vi "SetAxisParameter.vi"(8 "error in (no error)":errorcluster, 11 "ZanClass in":refnum<class "ZanClass.lvclass">) -> (0 "error out":errorcluster, 3 "ZanClass out":refnum<class "ZanClass.lvclass">)   [LabVIEW 2019, in "ZanClass.lvclass"]
uses:
  ZanClass.lvclass
  LLB/zmotion/zaux/zauxdll.lvlib
  Ctrl/CardTypr.ctl
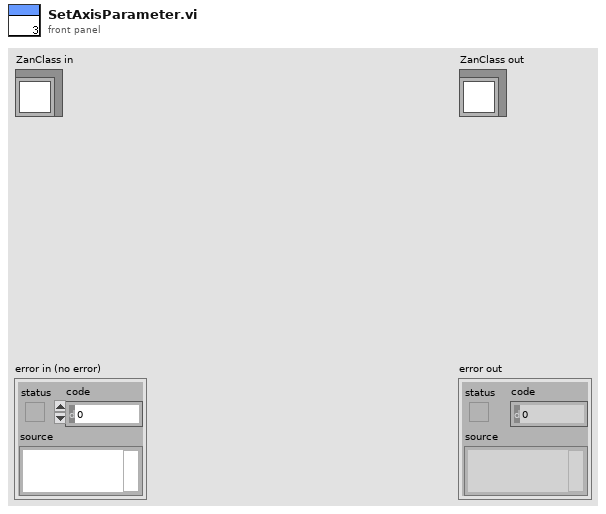
[diagram p1: front panel]
types:
  T1 = typedef "IO Card_Type.ctl" = enum16{"None", "Unidaq32", "6480", "2410C-64", "Zan", "DMC1000B", "16InOut", "Robot", "DMC3600"}
  T2 = cluster{"SetAType":i32, "SetUnit":sgl, "SetInvertStep":i32, "SetFwdIn":i32, "SetDatumIn":i32, "SetRevIn":i32, "SetAlmIn":i32}[]
  T3 = typedef "CardTypr.ctl" = enum16{"DMC2410", "DMC6480", "ZMotion", "KingServo RSCmd", "Zmotion2"}
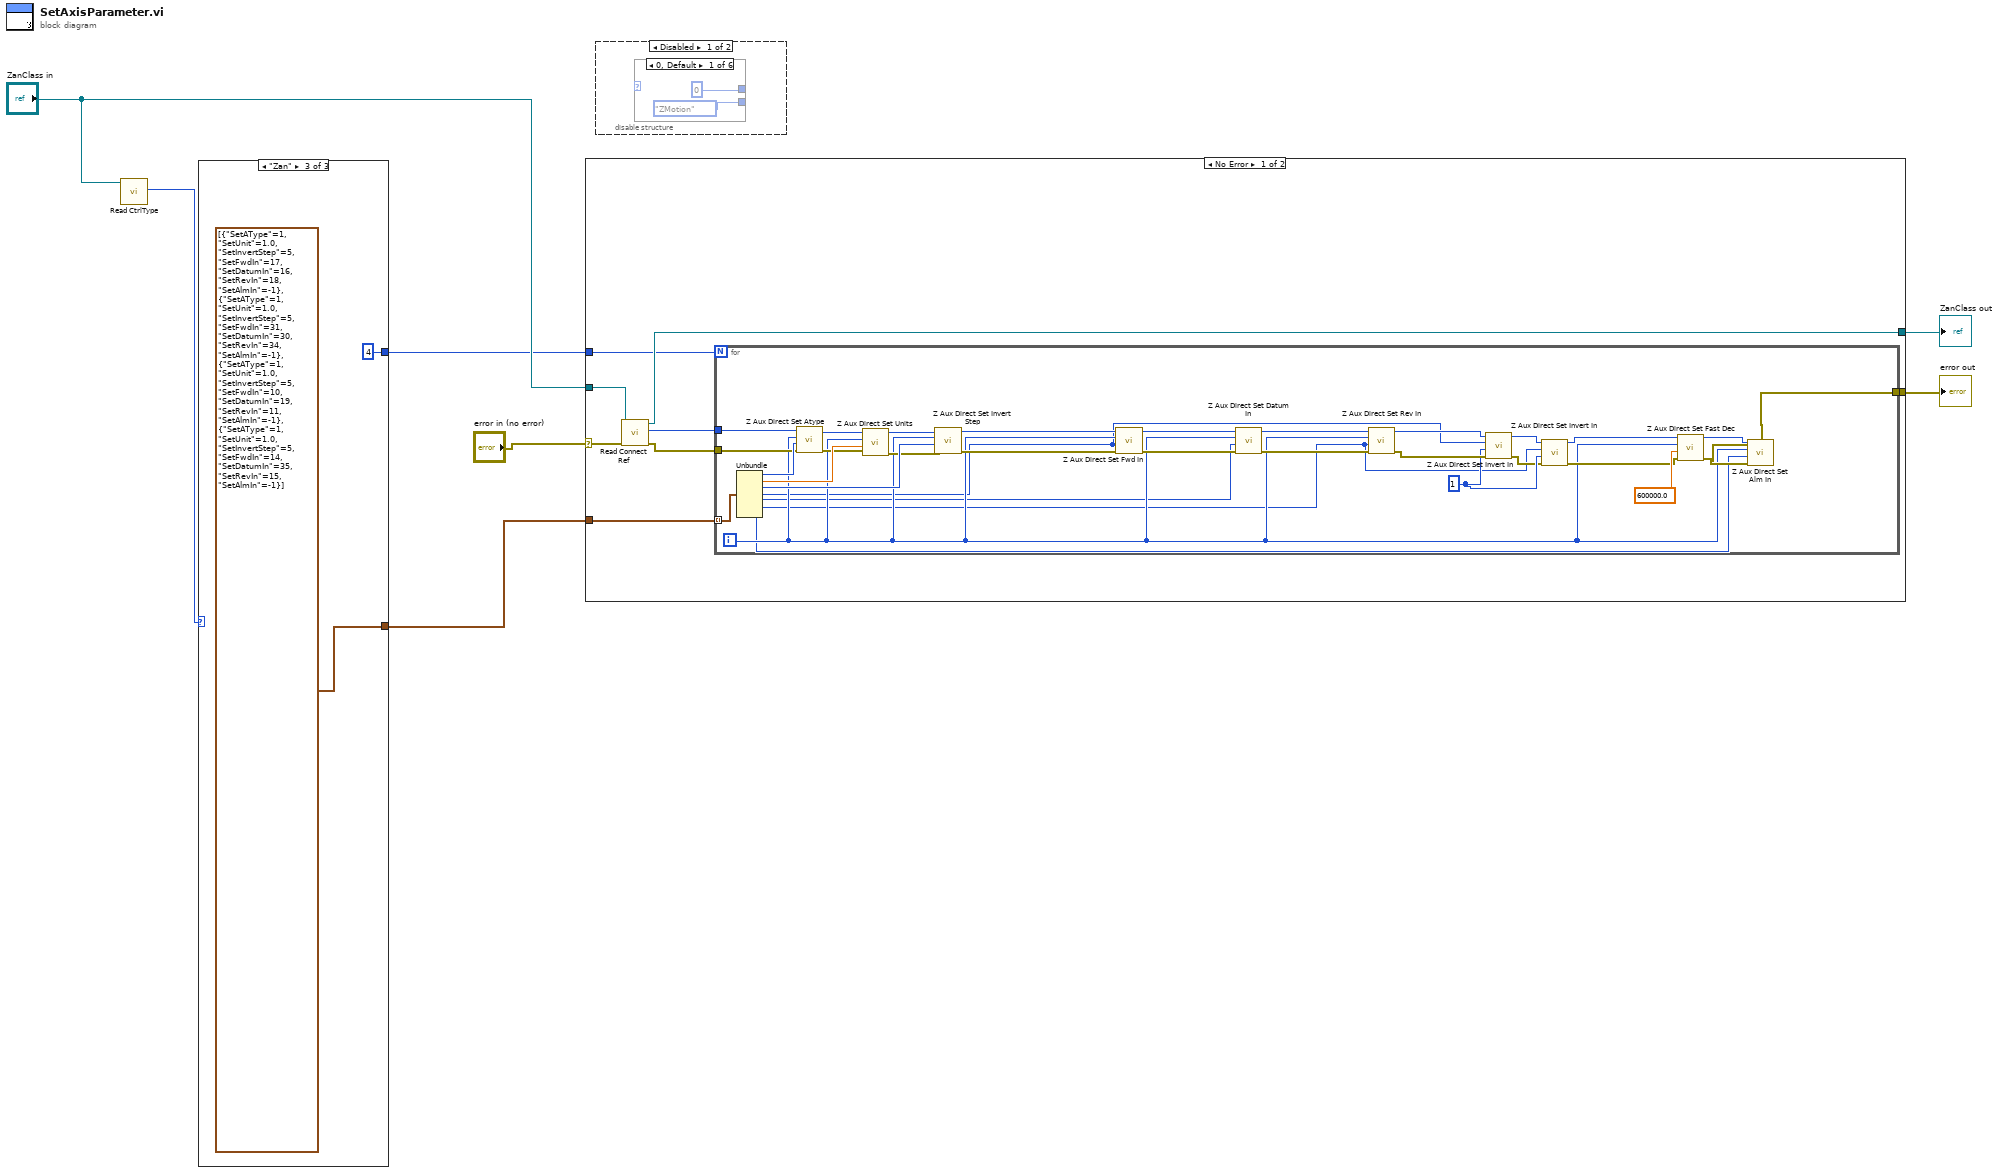
[diagram p0: block diagram]
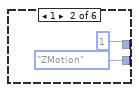
[diagram p2: hidden frame]
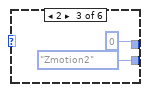
[diagram p3: hidden frame]
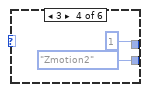
[diagram p4: hidden frame]
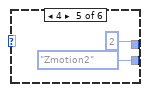
[diagram p5: hidden frame]
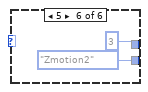
[diagram p6: hidden frame]
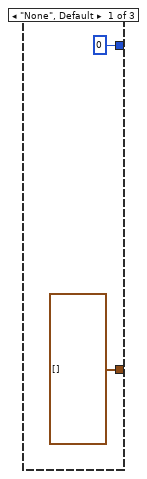
[diagram p8: hidden frame]
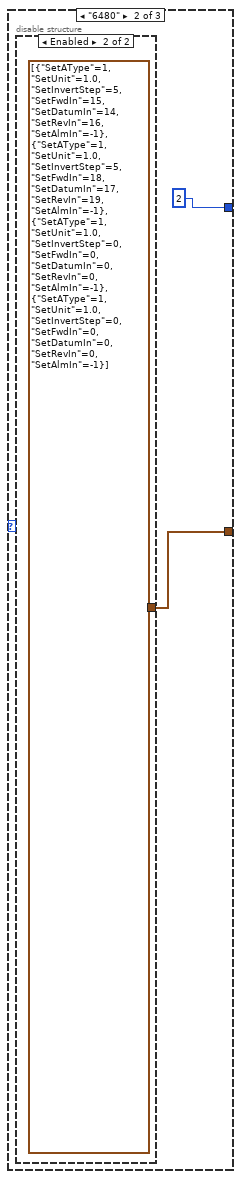
[diagram p9: hidden frame]
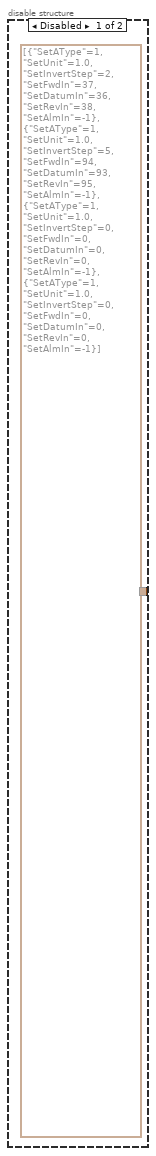
[diagram p10: hidden frame]
diagram:
  n1 = call-dynamic "Read CtrlType.vi"("AxisCard in"="ZanClass in") -> ("IO Card Type"=w2:T1)  [unwired: 8 in, 2 out]
  n2 = case shown="\"Zan\"" w2 {
    tunnel: [T2 [] w11 T2 [{"SetAType"=1, "SetUnit"=1.0, "SetInvertStep"=5, "SetFwdIn"=17, "SetDatumIn"=16, "SetRevIn"=18, "SetAlmIn"=-1}, {"SetAType"=1, "SetUnit"=1.0, "SetInvertStep"=5, "SetFwdIn"=31, "SetDatumIn"=30, "SetRevIn"=34, "SetAlmIn"=-1}, {"SetAType"=1, "SetUnit"=1.0, "SetInvertStep"=5, "SetFwdIn"=10, "SetDatumIn"=19, "SetRevIn"=11, "SetAlmIn"=-1}, {"SetAType"=1, "SetUnit"=1.0, "SetInvertStep"=5, "SetFwdIn"=14, "SetDatumIn"=35, "SetRevIn"=15, "SetAlmIn"=-1}]] -> w6
    tunnel: [0 2 4] -> w1
    frame "None", Default {
    }
    frame "6480" {
      n3 = disable-structure shown="Enabled" {
        disable-tunnel: [T2 [{"SetAType"=1, "SetUnit"=1.0, "SetInvertStep"=2, "SetFwdIn"=37, "SetDatumIn"=36, "SetRevIn"=38, "SetAlmIn"=-1}, {"SetAType"=1, "SetUnit"=1.0, "SetInvertStep"=5, "SetFwdIn"=94, "SetDatumIn"=93, "SetRevIn"=95, "SetAlmIn"=-1}, {"SetAType"=1, "SetUnit"=1.0, "SetInvertStep"=0, "SetFwdIn"=0, "SetDatumIn"=0, "SetRevIn"=0, "SetAlmIn"=-1}, {"SetAType"=1, "SetUnit"=1.0, "SetInvertStep"=0, "SetFwdIn"=0, "SetDatumIn"=0, "SetRevIn"=0, "SetAlmIn"=-1}] T2 [{"SetAType"=1, "SetUnit"=1.0, "SetInvertStep"=5, "SetFwdIn"=15, "SetDatumIn"=14, "SetRevIn"=16, "SetAlmIn"=-1}, {"SetAType"=1, "SetUnit"=1.0, "SetInvertStep"=5, "SetFwdIn"=18, "SetDatumIn"=17, "SetRevIn"=19, "SetAlmIn"=-1}, {"SetAType"=1, "SetUnit"=1.0, "SetInvertStep"=0, "SetFwdIn"=0, "SetDatumIn"=0, "SetRevIn"=0, "SetAlmIn"=-1}, {"SetAType"=1, "SetUnit"=1.0, "SetInvertStep"=0, "SetFwdIn"=0, "SetDatumIn"=0, "SetRevIn"=0, "SetAlmIn"=-1}]] -> w11
        frame Disabled {
        }
        frame Enabled {
        }
      }
    }
    frame "Zan" {
    }
  }
  n4 = case shown="No Error" "error in (no error)" {
    selector: "error in (no error)" -> [w19 w56]
    tunnel: "ZanClass in" -> [w23 w57]
    tunnel: w6 -> [w21 _]
    tunnel: [w20 w57] -> w5
    tunnel: [w17 w56] -> w4
    tunnel: w1 -> [w16 _]
    frame No Error {
      n5 = call-dynamic "Read Connect Ref.vi"("error in (no error)"=w19, "ZanClass in"=w23) -> ("error out"=w18:errorcluster, "CardHandle"=w22:i32, "ZanClass out"=w20:refnum<class "ZanClass.lvclass">)  [unwired: 6 in, 1 out]
      n6 = for {
        N: w16 -> [_]
        tunnel: w22 -> [w53]
        tunnel: w21 -> [w52] mode=indexing
        tunnel: w18 -> [w48]
        tunnel: [w37] -> w17
        i -> [w31]
        w34 = 1 ("bifInvert")
        n7 = Unbundle(w52) -> ("SetAType"=w51:i32, "SetUnit"=w50:sgl, "SetInvertStep"=w49:i32, "SetFwdIn"=w26:i32, "SetDatumIn"=w28:i32, "SetRevIn"=w25:i32, "SetAlmIn"=w27:i32)
        n8 = call "Z Aux Direct Set Atype.vi"("error in (no error)"=w48, "iValue"=w51, "iaxis"=w31, "handle"=w53) -> ("error out"=w47:errorcluster, "handle out"=w55:u32)  [unwired: 5 in, 1 out]
        n9 = call "Z Aux Direct Set Units.vi"("error in (no error)"=w47, "fValue"=w50, "iaxis"=w31, "handle"=w55) -> ("error out"=w46:errorcluster, "handle out"=w54:u32)  [unwired: 5 in, 1 out]
        n10 = call "Z Aux Direct Set Invert Step.vi"("error in (no error)"=w46, "iValue"=w49, "iaxis"=w31, "handle"=w54) -> ("error out"=w45:errorcluster, "handle out"=w32:u32)  [unwired: 5 in, 1 out]
        n11 = call "Z Aux Direct Set Fwd In.vi"("error in (no error)"=w45, "iValue"=w26, "iaxis"=w31, "handle"=w32) -> ("error out"=w44:errorcluster, "handle out"=w29:u32)  [unwired: 5 in, 1 out]
        n12 = call "Z Aux Direct Set Datum In.vi"("error in (no error)"=w44, "iValue"=w28, "iaxis"=w31, "handle"=w29) -> ("error out"=w43:errorcluster, "handle out"=w30:u32)  [unwired: 5 in, 1 out]
        n13 = call "Z Aux Direct Set Rev In.vi"("error in (no error)"=w43, "iValue"=w25, "iaxis"=w31, "handle"=w30) -> ("error out"=w41:errorcluster, "handle out"=w42:u32)  [unwired: 5 in, 1 out]
        n14 = call "Z Aux Direct Set Invert In.vi"("error in (no error)"=w41, "bifInvert"=w34, "ionum"=w26, "handle"=w42) -> ("error out"=w33:errorcluster, "handle out"=w24:u32)  [unwired: 5 in, 1 out]
        n15 = call "Z Aux Direct Set Invert In.vi"("error in (no error)"=w33, "bifInvert"=w34, "ionum"=w25, "handle"=w24) -> ("error out"=w35:errorcluster, "handle out"=w36:u32)  [unwired: 5 in, 1 out]
        n16 = call "Z Aux Direct Set Fast Dec.vi"("error in (no error)"=w35, "fValue"=sgl 600000.0, "iaxis"=w31, "handle"=w36) -> ("error out"=w38:errorcluster, "handle out"=w39:u32)  [unwired: 5 in, 1 out]
        n17 = call "Z Aux Direct Set Alm In.vi"("error in (no error)"=w38, "iValue"=w27, "iaxis"=w31, "handle"=w39) -> ("error out"=w37:errorcluster)  [unwired: 5 in, 2 out]
      }
    }
    frame Error {
    }
  }
  "error out" <- w4
  "ZanClass out" <- w5
  n18 = disable-structure shown="Disabled" {
    frame Disabled {
      n19 = case shown="0, Default" {
        selector: _ -> [_ _ _ _ _ _]
        tunnel: [CardTypr."ZMotion" ("CtrlType") CardTypr."ZMotion" ("CtrlType") CardTypr."Zmotion2" ("CtrlType") CardTypr."Zmotion2" ("CtrlType") CardTypr."Zmotion2" ("CtrlType") CardTypr."Zmotion2" ("CtrlType")] -> _
        tunnel: [0 1 0 1 2 3] -> _
        frame 0, Default {
        }
        frame 1 {
        }
        frame 2 {
        }
        frame 3 {
        }
        frame 4 {
        }
        frame 5 {
        }
      }
    }
    frame Enabled {
    }
  }
